vi "MyTest_noeudPython.vi"   [LabVIEW 2018]
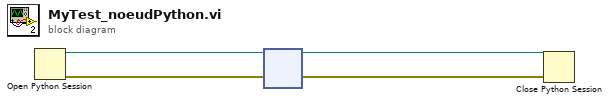
[diagram p0: block diagram]
diagram:
  n1 = Open Python Session() -> (session out=w4:refnum<k35>, error out=w3:errorcluster)  [unwired: 3 in]
  n2 = node(w4, w3) -> (w1:refnum<k35>, w2:errorcluster)  [unwired: 4 in, 2 out]
  n3 = Close Python Session(session in=w1, error in=w2) -> ()  [unwired: 1 out]
